vi "iFlex-Shutdown .vi"(4 "error in":errorcluster) -> (0 "error out":errorcluster)   [LabVIEW 2020]
uses:
  _Controls/iFlex.ctl
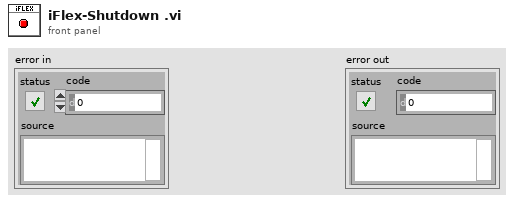
[diagram p1: front panel]
types:
  T1 = typedef "iFlex.ctl" = cluster{"561":dbl, "488":dbl, "Global Shutter":bool, "561 Shutter":bool}
  T2 = cluster{"iFlex Control":T1, "index of change":i32[]}
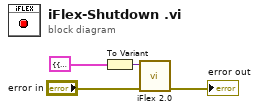
[diagram p0: block diagram]
diagram:
  n1 = To Variant(anything=T2 {"iFlex Control"={"561"=0.0, "488"=0.0, "Global Shutter"=FALSE, "561 Shutter"=FALSE}, "index of change"=[0, 1, 2, 3]}) -> (Variant=w4:variant)
  n2 = call "iFlex 2.0 .vi"("error in"="error in", "params"=w4) -> ("error out"=→"error out":errorcluster)  [unwired: 9 in]
